vi "getName.vi"() -> (3 "Name:":string)   [LabVIEW 2014]
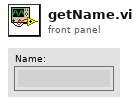
[diagram p1: front panel]
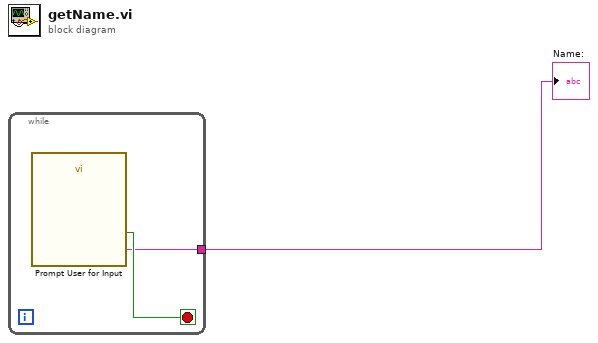
[diagram p0: block diagram]
diagram:
  n1 = while {
    tunnel: [w2] -> w1
    stop <- w3 stop-if-true
    n2 = call "Prompt User for Input"() -> ("Name:"=w2:string, "OK"=w3:bool)  [unwired: 17 in, 1 out]
  }
  "Name:" <- w1
